vi "LateralControl.vi"(6 "output range":cluster{"output high":dbl, "output low":dbl}, 7 "PID Gains lateral":T1={"proportional gain (Kc)"=0.008, "integral time (Ti, min)"=0.0, "derivative time (Td, min)"=-0.07}, 9 "Waypoint 0":dbl[](array[numeric]), 10 "Waypoint 1":dbl[](array[numeric]), 11 "Position":dbl[](array[numeric])) -> (1 "Numeric":dbl, 2 "y out":dbl, 3 "x out":dbl)   [LabVIEW 2017]
uses:
  <vilib>/Analysis/coordinate.llb/Wrap Angle (scalar).vi
  <vilib>/Analysis/coordinate.llb/2D Cartesian Coordinate Rotation (Scalar).vi
  <vilib>/Analysis/NI_AALPro.lvlib
  <vilib>/Analysis/NI_AAL_Angle.lvlib
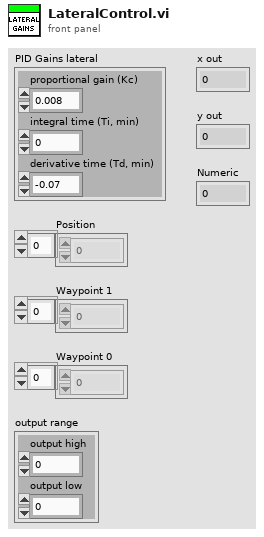
[diagram p1: front panel]
types:
  T1 = cluster{"proportional gain (Kc)":dbl, "integral time (Ti, min)":dbl, "derivative time (Td, min)":dbl}
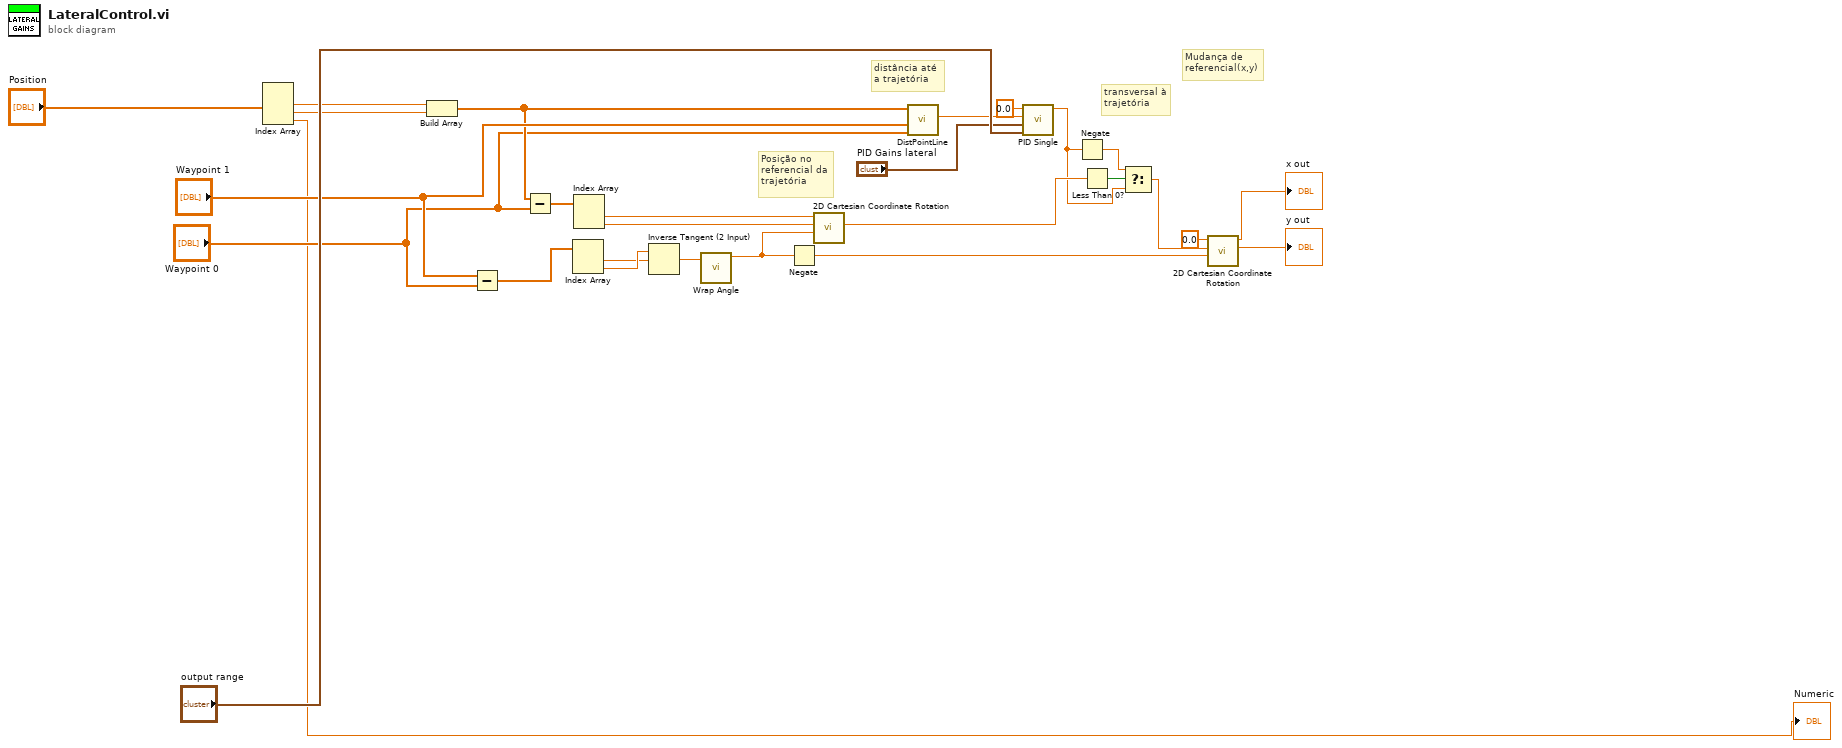
[diagram p0: block diagram]
diagram:
  # "Posição no \nreferencial da\ntrajetória"
  # "distância até \na trajetória"
  # "Mudança de \nreferencial(x,y)"
  # "transversal à\ntrajetória"
  n1 = Index Array(array="Position") -> (element #1=w8:dbl, element #2=w9:dbl, element #3=→"Numeric":dbl)  [unwired: 3 in]
  n2 = Build Array(w8, w9) -> (w23:dbl[])
  n3 = Subtract(x="Waypoint 1", y="Waypoint 0") -> (x-y=w19:dbl[])
  n4 = Subtract(x=w23, y="Waypoint 0") -> (x-y=w14:dbl[])
  n5 = Index Array(array=w19) -> (element #1=w6:dbl, element #2=w20:dbl)  [unwired: 2 in]
  n6 = Index Array(array=w14) -> (element #1=w15:dbl, element #2=w16:dbl)  [unwired: 2 in]
  n7 = Inverse Tangent (2 Input)(1:w6, 2:w20) -> (0:w7:dbl)
  n8 = call-poly <vilib>:"Wrap Angle.vi"("angle in"=w7) -> ("angle out"=w22:dbl)  [unwired: 9 in, 1 out]
  n9 = Negate(x=w22) -> (-x=w5:dbl)
  n10 = call-poly <vilib>:"2D Cartesian Coordinate Rotation.vi"("theta"=w22, "y"=w16, "x"=w15) -> ("y out"=w13:dbl)  [unwired: 6 in, 2 out]
  n11 = call "DistPointLine.vi"("P2"="Waypoint 0", "P1"="Waypoint 1", "Q"=w23) -> ("distance"=w2:dbl)  [unwired: 8 in]
  n12 = call "PID Single.vi"("Limits"="output range", "PID gains in"="PID Gains lateral", "Variable"=w2, "Setpoint"=0.0) -> ("Out"=w11:dbl)  [unwired: 7 in]
  n13 = Negate(x=w11) -> (-x=w10:dbl)
  n14 = Less Than 0?(x=w13) -> (x < 0?=w17:bool)
  n15 = Select(t=w10, s=w17, f=w11) -> (s? t:f=w12:dbl)
  n16 = call-poly <vilib>:"2D Cartesian Coordinate Rotation.vi"("theta"=w5, "y"=w12, "x"=0.0) -> ("y out"=→"y out":dbl, "x out"=→"x out":dbl)  [unwired: 6 in, 1 out]
